vi "VI Tree.vi"   [LabVIEW 2010, in "Agilent 3458.lvlib"]
doc: "This is the instrument driver for the AG 3458A. The VI Tree displays all the user-callable VIs of the instrument driver in an organized table."
uses:
  <instrlib>/Agilent 3458/Agilent 3458.lvlib
  <instrlib>/Agilent 3458/Public/Data/Read Measurement(Single Point).vi
  <instrlib>/Agilent 3458/Public/Data/Low Level/Fetch Measurement(Single Point).vi
panel:
  # "© 2007 National Instruments.  ALL RIGHTS RESERVED."
  # "SEE DIAGRAM\nFOR VI TREE."
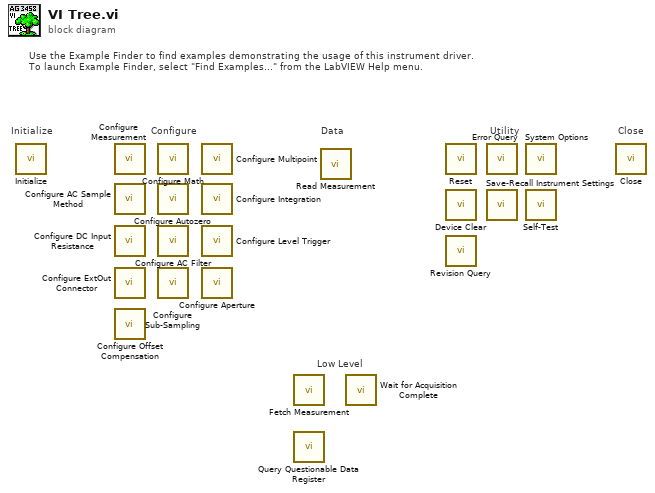
[diagram p0: block diagram]
diagram:
  # "Low Level"
  # "Use the Example Finder to find examples demonstrating the usage of this instrument driver.\nTo launch Example Finder, select \"Find Examples...\" from the LabVIEW Help menu."
  # "Configure"
  # "Utility"
  # "Data"
  # "Close"
  # "Initialize"
  n1 = call <instrlib>:"Initialize.vi"() -> ()  [unwired: 10 in, 2 out]
  n2 = call <instrlib>:"Configure Measurement.vi"() -> ()  [unwired: 14 in, 2 out]
  n3 = call <instrlib>:"Configure AC Sample Method.vi"() -> ()  [unwired: 10 in, 2 out]
  n4 = call <instrlib>:"Configure DC Input Resistance.vi"() -> ()  [unwired: 10 in, 2 out]
  n5 = call <instrlib>:"Configure ExtOut Connector.vi"() -> ()  [unwired: 10 in, 2 out]
  n6 = call <instrlib>:"Configure Offset Compensation.vi"() -> ()  [unwired: 10 in, 2 out]
  n7 = call <instrlib>:"Configure Math.vi"() -> ()  [unwired: 14 in, 2 out]
  n8 = call <instrlib>:"Configure Autozero.vi"() -> ()  [unwired: 10 in, 2 out]
  n9 = call <instrlib>:"Configure AC Filter.vi"() -> ()  [unwired: 10 in, 2 out]
  n10 = call <instrlib>:"Configure Sub-Sampling.vi"() -> ()  [unwired: 10 in, 2 out]
  n11 = call <instrlib>:"Configure Multipoint.vi"() -> ()  [unwired: 10 in, 2 out]
  n12 = call <instrlib>:"Configure Integration.vi"() -> ()  [unwired: 10 in, 2 out]
  n13 = call <instrlib>:"Configure Level Trigger.vi"() -> ()  [unwired: 10 in, 2 out]
  n14 = call <instrlib>:"Configure Aperture.vi"() -> ()  [unwired: 10 in, 2 out]
  n15 = call-poly <instrlib>:"Fetch Measurement.vi"() -> ()  [unwired: 13 in, 3 out]
  n16 = call <instrlib>:"Query Questionable Data Register.vi"() -> ()  [unwired: 9 in, 3 out]
  n17 = call-poly <instrlib>:"Read Measurement.vi"() -> ()  [unwired: 13 in, 3 out]
  n18 = call <instrlib>:"Wait for Acquisition Complete.vi"() -> ()  [unwired: 10 in, 2 out]
  n19 = call <instrlib>:"Reset.vi"() -> ()  [unwired: 10 in, 2 out]
  n20 = call <instrlib>:"Device Clear.vi"() -> ()  [unwired: 10 in, 2 out]
  n21 = call <instrlib>:"Revision Query.vi"() -> ()  [unwired: 7 in, 5 out]
  n22 = call <instrlib>:"Error Query.vi"() -> ()  [unwired: 8 in, 4 out]
  n23 = call <instrlib>:"Save-Recall Instrument Settings.vi"() -> ()  [unwired: 10 in, 2 out]
  n24 = call <instrlib>:"System Options.vi"() -> ()  [unwired: 10 in, 2 out]
  n25 = call <instrlib>:"Self-Test.vi"() -> ()  [unwired: 10 in, 2 out]
  n26 = call <instrlib>:"Close.vi"() -> ()  [unwired: 11 in, 1 out]
